vi "Plan_writer.vi"(7 "Enum":enum16{"SECTION1", "SECTION2"}(ring)=enum."SECTION2", 11 "SECTION IN":T1={"FG CAT NO"="AUF3C200601", "HAUSING"="", "DOOR 1 STATUS"="PENDING", "PMR"="", "DOOR 2 STATUS"="PENDING", "MAGNETIC AS"="", "DOOR 3 STATUS"="PENDING", "CBCT"="", "DOOR 4 STATUS"="PENDING", "KINAMETIC AS"="", "DOOR 9 STATUS"="PENDING", "REGISTOR 1"="", "DOOR 10 STATUS"="PENDING", "QUANTITY"=80}) -> (2 "Section Second 45":string[](array[string]), 3 "Section first 45":string[](array[string]))   [LabVIEW 2017]
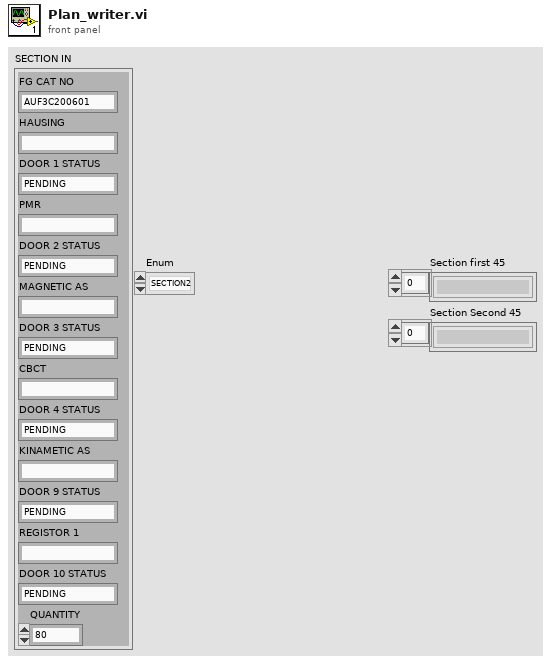
[diagram p1: front panel]
types:
  T1 = cluster{"FG CAT NO":string, "HAUSING":string, "DOOR 1 STATUS":string, "PMR":string, "DOOR 2 STATUS":string, "MAGNETIC AS":string, "DOOR 3 STATUS":string, "CBCT":string, "DOOR 4 STATUS":string, "KINAMETIC AS":string, "DOOR 9 STATUS":string, "REGISTOR 1":string, "DOOR 10 STATUS":string, "QUANTITY":u16}
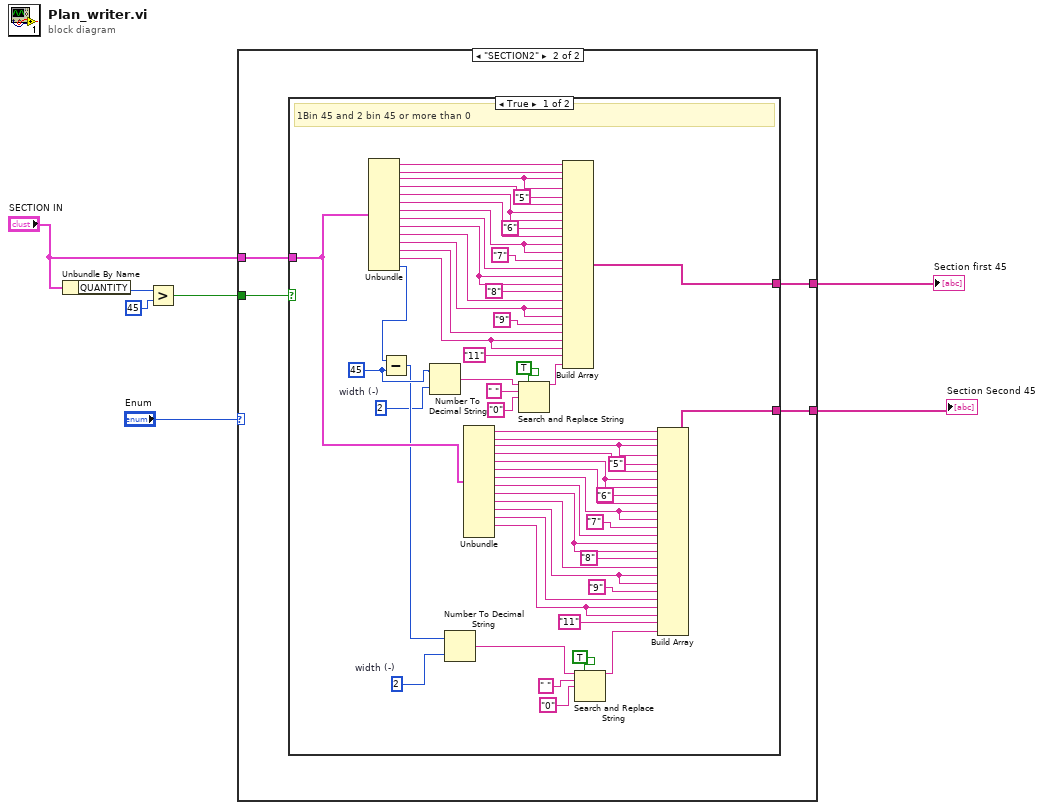
[diagram p0: block diagram]
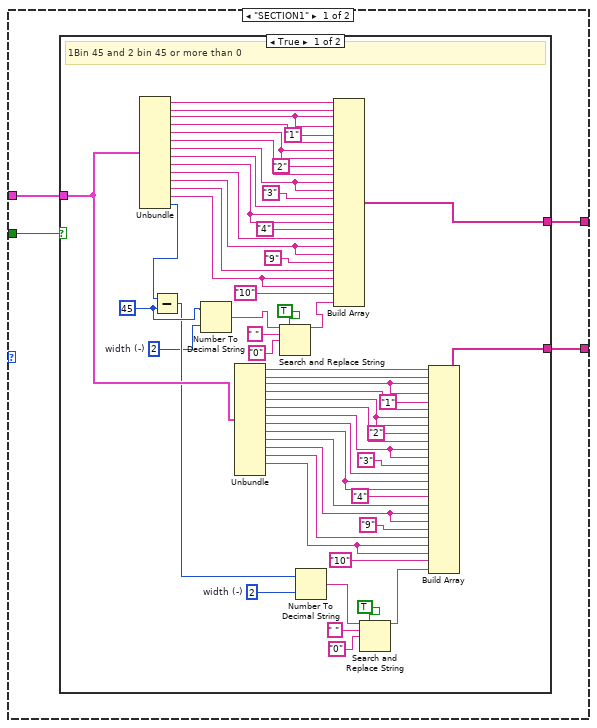
[diagram p2: hidden frame]
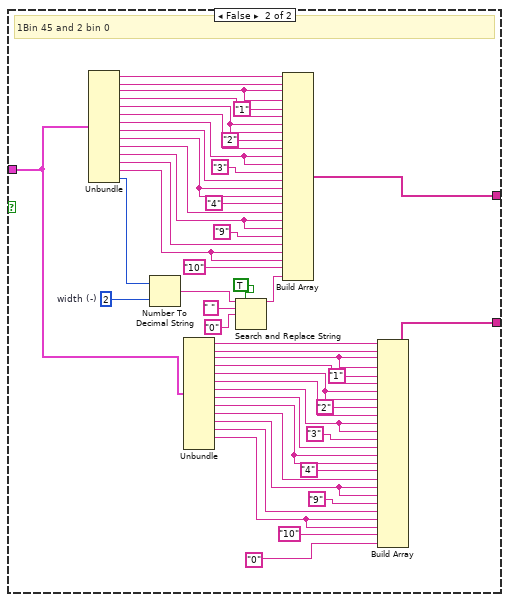
[diagram p3: hidden frame]
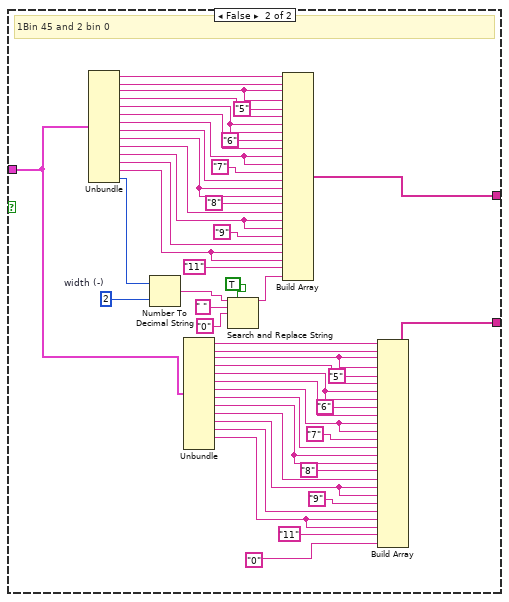
[diagram p4: hidden frame]
diagram:
  n1 = Unbundle By Name("SECTION IN") -> ("QUANTITY"=w5:u16)
  n2 = Greater?(x=w5, y=u16 45) -> (0:w4:bool)
  n3 = case shown="\"SECTION2\"" "Enum" {
    tunnel: "SECTION IN" -> [w11 w120]
    tunnel: w4 -> [w10 w119]
    tunnel: [w9 w118] -> w3
    tunnel: [w8 w117] -> w2
    frame "SECTION1" {
      n4 = case shown="True" w10 {
        tunnel: w11 -> [w26 w77]
        tunnel: [w52 w103] -> w9
        tunnel: [w25 w76] -> w8
        frame True {
          w14 = i16 2  # width (-)
          w15 = i16 2  # width (-)
          w53 = u16 45
          # "1Bin 45 and 2 bin 45 or more than 0"
          n5 = Unbundle(w26) -> ("FG CAT NO"=w67:string, "HAUSING"=w66:string, "DOOR 1 STATUS"=w65:string, "PMR"=w64:string, "DOOR 2 STATUS"=w63:string, "MAGNETIC AS"=w62:string, "DOOR 3 STATUS"=w61:string, "CBCT"=w60:string, "DOOR 4 STATUS"=w59:string, "KINAMETIC AS"=w58:string, "DOOR 9 STATUS"=w57:string, "REGISTOR 1"=w56:string, "DOOR 10 STATUS"=w55:string, "QUANTITY"=w54:u16)
          n6 = Subtract(x=w54, y=w53) -> (x-y=w24:u16)
          n7 = Number To Decimal String(number=w53, width (-)=w14) -> (decimal integer string=w13:string)
          n8 = Unbundle(w26) -> ("FG CAT NO"=w27:string, "HAUSING"=w28:string, "DOOR 1 STATUS"=w29:string, "PMR"=w30:string, "DOOR 2 STATUS"=w31:string, "MAGNETIC AS"=w32:string, "DOOR 3 STATUS"=w33:string, "CBCT"=w34:string, "DOOR 4 STATUS"=w35:string, "KINAMETIC AS"=w36:string, "DOOR 9 STATUS"=w37:string, "REGISTOR 1"=w38:string, "DOOR 10 STATUS"=w39:string)  [unwired: 1 out]
          n9 = Search and Replace String(replace all?=TRUE ("replace all? (F)"), input string=w13, search string=" ", replace string="0") -> (result string=w12:string)  [unwired: 4 in, 3 out]
          n10 = Number To Decimal String(number=w24, width (-)=w15) -> (decimal integer string=w16:string)
          n11 = Build Array(w67, w66, w65, w65, "1", w64, w63, w63, "2", w62, w61, w61, "3", w60, w59, w59, "4", w58, w57, w57, "9", w56, w55, w55, "10", w12) -> (w52:string[])
          n12 = Search and Replace String(replace all?=TRUE ("replace all? (F)"), input string=w16, search string=" ", replace string="0") -> (result string=w17:string)  [unwired: 4 in, 3 out]
          n13 = Build Array(w27, w28, w29, w29, "1", w30, w31, w31, "2", w32, w33, w33, "3", w34, w35, w35, "4", w36, w37, w37, "9", w38, w39, w39, "10", w17) -> (w25:string[])
        }
        frame False {
          w68 = i16 2  # width (-)
          # "1Bin 45 and 2 bin 0"
          n14 = Unbundle(w77) -> ("FG CAT NO"=w116:string, "HAUSING"=w115:string, "DOOR 1 STATUS"=w114:string, "PMR"=w113:string, "DOOR 2 STATUS"=w112:string, "MAGNETIC AS"=w111:string, "DOOR 3 STATUS"=w110:string, "CBCT"=w109:string, "DOOR 4 STATUS"=w108:string, "KINAMETIC AS"=w107:string, "DOOR 9 STATUS"=w106:string, "REGISTOR 1"=w105:string, "DOOR 10 STATUS"=w104:string, "QUANTITY"=w74:u16)
          n15 = Number To Decimal String(number=w74, width (-)=w68) -> (decimal integer string=w70:string)
          n16 = Unbundle(w77) -> ("FG CAT NO"=w78:string, "HAUSING"=w79:string, "DOOR 1 STATUS"=w80:string, "PMR"=w81:string, "DOOR 2 STATUS"=w82:string, "MAGNETIC AS"=w83:string, "DOOR 3 STATUS"=w84:string, "CBCT"=w85:string, "DOOR 4 STATUS"=w86:string, "KINAMETIC AS"=w87:string, "DOOR 9 STATUS"=w88:string, "REGISTOR 1"=w89:string, "DOOR 10 STATUS"=w90:string)  [unwired: 1 out]
          n17 = Search and Replace String(replace all?=TRUE ("replace all? (F)"), input string=w70, search string=" ", replace string="0") -> (result string=w69:string)  [unwired: 4 in, 3 out]
          n18 = Build Array(w116, w115, w114, w114, "1", w113, w112, w112, "2", w111, w110, w110, "3", w109, w108, w108, "4", w107, w106, w106, "9", w105, w104, w104, "10", w69) -> (w103:string[])
          n19 = Build Array(w78, w79, w80, w80, "1", w81, w82, w82, "2", w83, w84, w84, "3", w85, w86, w86, "4", w87, w88, w88, "9", w89, w90, w90, "10", "0") -> (w76:string[])
        }
      }
    }
    frame "SECTION2" {
      n20 = case shown="True" w119 {
        tunnel: w120 -> [w135 w186]
        tunnel: [w161 w212] -> w118
        tunnel: [w134 w185] -> w117
        frame True {
          w131 = i16 2  # width (-)
          w132 = i16 2  # width (-)
          w162 = u16 45
          # "1Bin 45 and 2 bin 45 or more than 0"
          n21 = Unbundle(w135) -> ("FG CAT NO"=w176:string, "HAUSING"=w175:string, "DOOR 1 STATUS"=w174:string, "PMR"=w173:string, "DOOR 2 STATUS"=w172:string, "MAGNETIC AS"=w171:string, "DOOR 3 STATUS"=w170:string, "CBCT"=w169:string, "DOOR 4 STATUS"=w168:string, "KINAMETIC AS"=w167:string, "DOOR 9 STATUS"=w166:string, "REGISTOR 1"=w165:string, "DOOR 10 STATUS"=w164:string, "QUANTITY"=w163:u16)
          n22 = Subtract(x=w163, y=w162) -> (x-y=w133:u16)
          n23 = Number To Decimal String(number=w162, width (-)=w131) -> (decimal integer string=w121:string)
          n24 = Number To Decimal String(number=w133, width (-)=w132) -> (decimal integer string=w127:string)
          n25 = Unbundle(w135) -> ("FG CAT NO"=w136:string, "HAUSING"=w137:string, "DOOR 1 STATUS"=w138:string, "PMR"=w139:string, "DOOR 2 STATUS"=w140:string, "MAGNETIC AS"=w141:string, "DOOR 3 STATUS"=w142:string, "CBCT"=w143:string, "DOOR 4 STATUS"=w144:string, "KINAMETIC AS"=w145:string, "DOOR 9 STATUS"=w146:string, "REGISTOR 1"=w147:string, "DOOR 10 STATUS"=w148:string)  [unwired: 1 out]
          n26 = Search and Replace String(replace all?=TRUE ("replace all? (F)"), input string=w121, search string=" ", replace string="0") -> (result string=w122:string)  [unwired: 4 in, 3 out]
          n27 = Build Array(w176, w175, w174, w174, "5", w173, w172, w172, "6", w171, w170, w170, "7", w169, w168, w168, "8", w167, w166, w166, "9", w165, w164, w164, "11", w122) -> (w161:string[])
          n28 = Search and Replace String(replace all?=TRUE ("replace all? (F)"), input string=w127, search string=" ", replace string="0") -> (result string=w126:string)  [unwired: 4 in, 3 out]
          n29 = Build Array(w136, w137, w138, w138, "5", w139, w140, w140, "6", w141, w142, w142, "7", w143, w144, w144, "8", w145, w146, w146, "9", w147, w148, w148, "11", w126) -> (w134:string[])
        }
        frame False {
          w177 = i16 2  # width (-)
          # "1Bin 45 and 2 bin 0"
          n30 = Unbundle(w186) -> ("FG CAT NO"=w225:string, "HAUSING"=w224:string, "DOOR 1 STATUS"=w223:string, "PMR"=w222:string, "DOOR 2 STATUS"=w221:string, "MAGNETIC AS"=w220:string, "DOOR 3 STATUS"=w219:string, "CBCT"=w218:string, "DOOR 4 STATUS"=w217:string, "KINAMETIC AS"=w216:string, "DOOR 9 STATUS"=w215:string, "REGISTOR 1"=w214:string, "DOOR 10 STATUS"=w213:string, "QUANTITY"=w183:u16)
          n31 = Number To Decimal String(number=w183, width (-)=w177) -> (decimal integer string=w178:string)
          n32 = Unbundle(w186) -> ("FG CAT NO"=w187:string, "HAUSING"=w188:string, "DOOR 1 STATUS"=w189:string, "PMR"=w190:string, "DOOR 2 STATUS"=w191:string, "MAGNETIC AS"=w192:string, "DOOR 3 STATUS"=w193:string, "CBCT"=w194:string, "DOOR 4 STATUS"=w195:string, "KINAMETIC AS"=w196:string, "DOOR 9 STATUS"=w197:string, "REGISTOR 1"=w198:string, "DOOR 10 STATUS"=w199:string)  [unwired: 1 out]
          n33 = Search and Replace String(replace all?=TRUE ("replace all? (F)"), input string=w178, search string=" ", replace string="0") -> (result string=w179:string)  [unwired: 4 in, 3 out]
          n34 = Build Array(w225, w224, w223, w223, "5", w222, w221, w221, "6", w220, w219, w219, "7", w218, w217, w217, "8", w216, w215, w215, "9", w214, w213, w213, "11", w179) -> (w212:string[])
          n35 = Build Array(w187, w188, w189, w189, "5", w190, w191, w191, "6", w192, w193, w193, "7", w194, w195, w195, "8", w196, w197, w197, "9", w198, w199, w199, "11", "0") -> (w185:string[])
        }
      }
    }
  }
  "Section first 45" <- w3
  "Section Second 45" <- w2
